vi "Read Lockin Parameters.vi"(0 "tdms file":refnum<k34>, 5 "group name in":string, 9 "Channel name":string, 11 "Error In":errorcluster, 12 "Lockin parameters":T1={"Frequency"=0.0, "Phase"=0.0, "Syncronous"=FALSE, "Points per sine wave"=0, "DDS"=FALSE, "Frequency word"=0, "Phase word"=0, "DDS modulus"=15120, "DDS clock"=125000000.0} {"DDS clock" format="%_17pHz"; "DDS modulus" format="0x%x (%d)"; "Phase" format="%#_gdeg"; "Frequency" format="%_17pHz"}) -> (2 "dt":dbl, 4 "tdms file out":refnum<k34>, 8 "t0":timestamp, 10 "Channel length":u64, 14 "Lockin parameters out":T1={"Frequency"=0.0, "Phase"=0.0, "Syncronous"=FALSE, "Points per sine wave"=0, "DDS"=FALSE, "Frequency word"=0, "Phase word"=0, "DDS modulus"=15120, "DDS clock"=125000000.0} {"DDS clock" format="%_17pHz"; "DDS modulus" format="0x%x (%d)"; "Phase" format="%#_gdeg"; "Frequency" format="%_17pHz"}, 15 "Error Out":errorcluster)   [LabVIEW 2016]
uses:
  Lockin Parameters.ctl
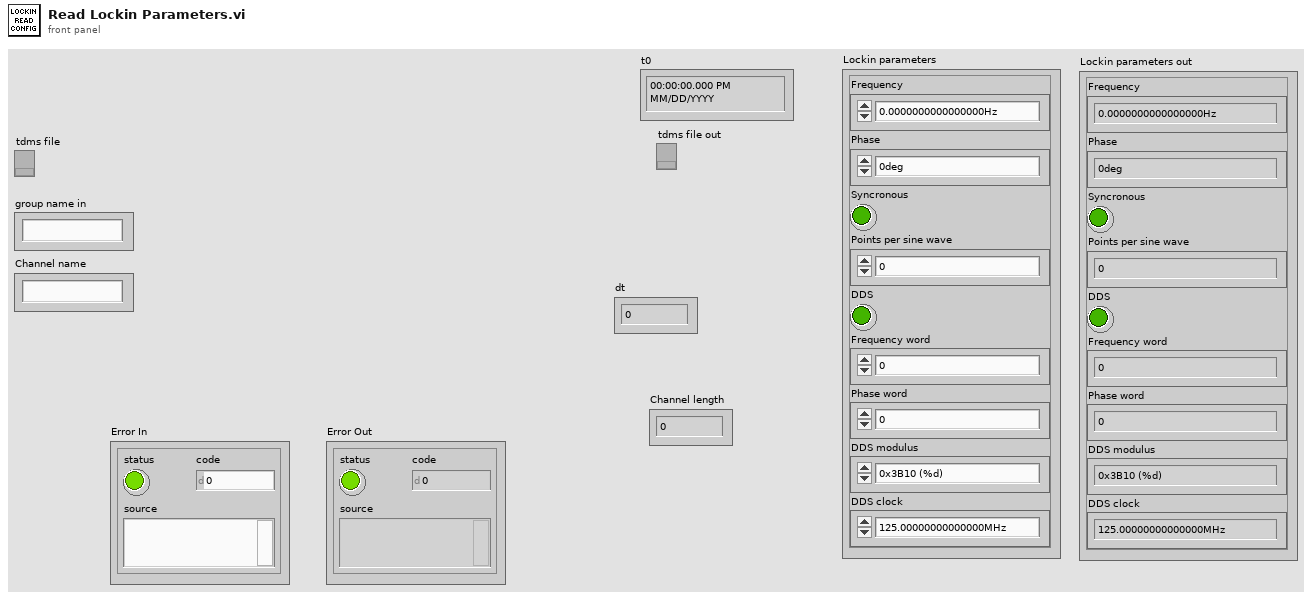
[diagram p1: front panel]
types:
  T1 = typedef "Lockin Parameters.ctl" = cluster{"Frequency":dbl, "Phase":dbl, "Syncronous":bool, "Points per sine wave":i32, "DDS":bool, "Frequency word":u32, "Phase word":u32, "DDS modulus":i64, "DDS clock":dbl}
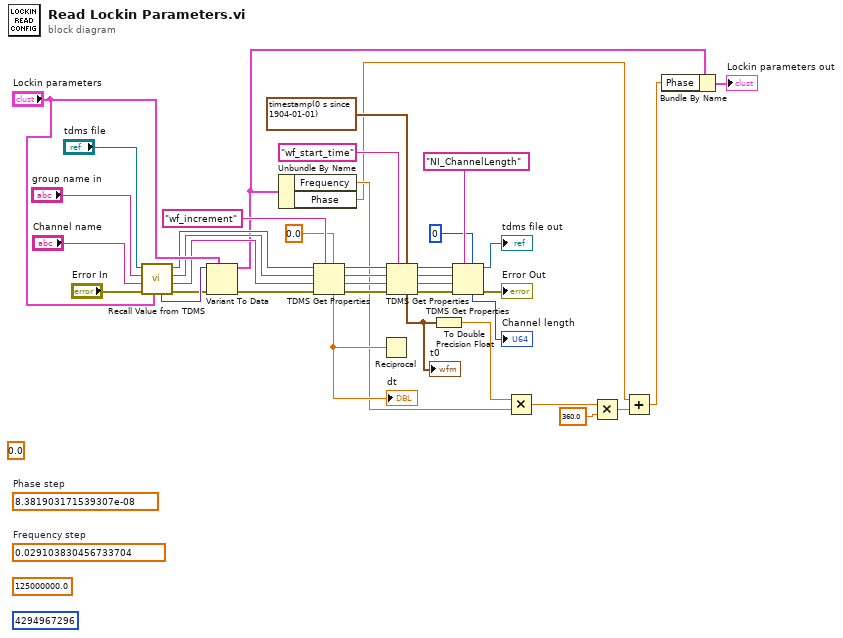
[diagram p0: block diagram]
diagram:
  (unwired) 0.0 ("index")
  (unwired) 8.381903171539307e-08  # Phase step
  (unwired) 0.029103830456733704  # Frequency step
  (unwired) u64 4294967296
  (unwired) 125000000.0
  n1 = call "Recall Value from TDMS.vi"("Value"="Lockin parameters", "Error In"="Error In", "channel name"="Channel name", "group name"="group name in", "tdms file"="tdms file") -> ("Error Out"=w23:errorcluster, "channel name out"=w15:string, "group name out"=w16:string, "tdms file out"=w21:refnum<k34>, "Value out"=w25:variant)  [unwired: 2 in]
  n2 = Variant To Data(error in=w23, type="Lockin parameters", Variant=w25) -> (data=w14:T1, error out=w17:errorcluster)
  n3 = Unbundle By Name(w14) -> ("Frequency"=w13:dbl, "Phase"=w12:dbl)
  n4 = TDMS Get Properties(5:0.0, 7:"wf_increment", 8:w17, 9:w15, 10:w16, 11:w21) -> (0:w37:errorcluster, 1:w34:string, 2:w35:string, 3:w36:refnum<k34>, 4:w30:dbl)  [unwired: 1 out]
  "dt" <- w30
  n5 = Reciprocal(x=w30) -> ()  [unwired: 1 out]
  n6 = TDMS Get Properties(5:timestamp(0 s since 1904-01-01) ("t0"), 7:"wf_start_time", 8:w37, 9:w34, 10:w35, 11:w36) -> (0:w3:errorcluster, 1:w4:string, 2:w5:string, 3:w7:refnum<k34>, 4:w31:timestamp)  [unwired: 1 out]
  "t0" <- w31
  n7 = To Double Precision Float(number=w31) -> (double precision float=w29:dbl)
  n8 = TDMS Get Properties(5:u64 0, 7:"NI_ChannelLength" ("property name"), 8:w3, 9:w4, 10:w5, 11:w7) -> (0:→"Error Out":errorcluster, 3:→"tdms file out":refnum<k34>, 4:→"Channel length":u64)  [unwired: 3 out]
  n9 = Multiply(x=w29, y=w13) -> (x*y=w27:dbl)
  n10 = Multiply(x=w27, y=360.0) -> (x*y=w26:dbl)
  n11 = Add(x=w12, y=w26) -> (x+y=w10:dbl)
  n12 = Bundle By Name(cluster=w14, "Phase"=w10) -> (→"Lockin parameters out":T1)
